vi "mod_Rayleigh Selective Fading (Gans).vi"(0 "profile length (samples)":i32=1000, 1 "number of paths":i32, 5 "sampling frequency (Hz)":dbl=1.0 format="%.2f", 7 "doppler spread (Hz)":dbl=0.01 format="%.2p", 9 "seed in (0xFFFFFFFF)":i32=-1 format="%.0x", 11 "error in (no error)":errorcluster, 12 "fading variance":dbl=1.0 format="%.2f", 13 "reset? (T)":bool=TRUE) -> (4 "Rayleigh fading profile":cdb[][](array[numeric]), 10 "seed out":i32 format="%.0x", 15 "error out":errorcluster)   [LabVIEW 2020, in "niDMT.lvlib"]
doc: "The Rayleigh fading channel is generated based on Clarke and Gans Model using the Doppler filter with U-shaped power spectral density. \n \n\n Inputs:\n 1) Doppler spread (Hz) \n - range : double precision (default:20)\n - an example : a running vehicle with 65mph (104km/h), the carrier frequency of 900MHz\n The speed of the vehicle = 65*1.6*1000/3600 = 28.89m/s\n Doppler frequency = (900MHz)*(28.89m/s)/(300*10^6m/s) = 86.67 Hz\n 2) Fading variance : the variance of the fading channel output\n - range : double precision (default:2)\n 3) Input waveform : Input signal samples\n - some default values were set.\n (dt:0.00025, the number of samples:4000)\n 4) seed in (0xFFFFFFFF)\n 5) Error in\n\n Outputs:\n 1) Rayleigh fading profile : the complex fading channel output\n 2) Error out"
uses:
  <vilib>/addons/Modulation/niDMT.lvlib
  <vilib>/addons/Modulation/niAMT.lvlib
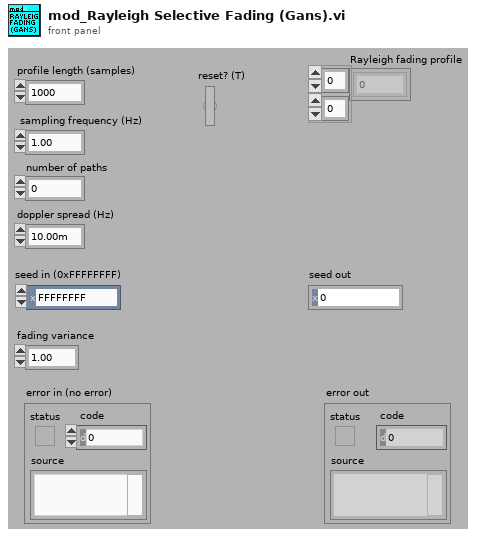
[diagram p1: front panel]
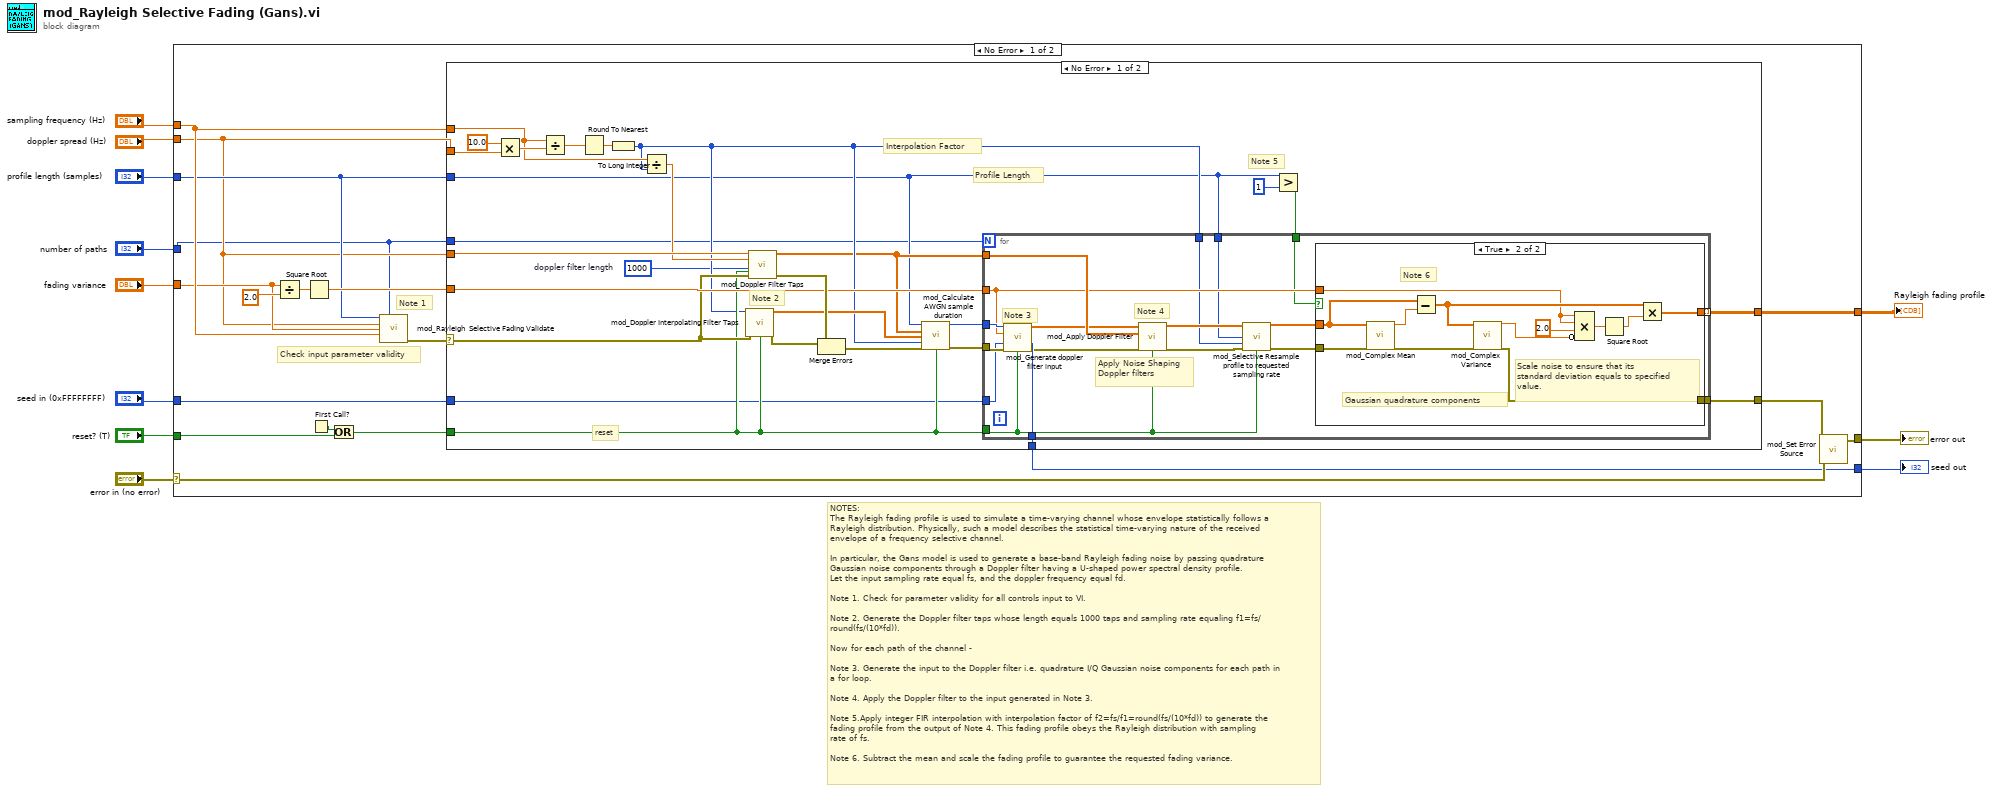
[diagram p0: block diagram]
diagram:
  # "NOTES:\nThe Rayleigh fading profile is used to simulate a time-varying channel whose envelope statistically follows a Rayleigh distribution. Physically, such a model describes the statistical time-varying nature of the received envelope of a frequency selective channel.\n\t\t  \nIn particular, the Gans model is used to generate a base-band Rayleigh fading noise by passing quadrature Gaussian noise components through a Doppler filter having a U-shaped power spectral density profile. \nLet the input sampling rate equal fs, and the doppler frequency equal fd.\n\nNote 1. Check for parameter validity for all controls input to VI.\n\nNote 2. Generate the Doppler filter taps whose length equals 1000 taps and sampling rate equaling f1=fs/round(fs/(10*fd)).\n\nNow for each path of the channel -\n\nNote 3. Generate the input to the Doppler filter i.e. quadrature I/Q Gaussian noise components for each path in a for loop.\n\nNote 4. Apply the Doppler filter to the input generated in Note 3.\n\nNote 5.Apply integer FIR interpolation with interpolation factor of f2=fs/f1=round(fs/(10*fd)) to generate the fading profile from the output of Note 4. This fading profile obeys the Rayleigh distribution with sampling\nrate of fs. \n\nNote 6. Subtract the mean and scale the fading profile to guarantee the requested fading variance."
  n1 = case shown="No Error" "error in (no error)" {
    selector: "error in (no error)" -> [w27 w91]
    tunnel: [w28 w91] -> w11
    tunnel: [w29 _] -> w2
    tunnel: "sampling frequency (Hz)" -> [w19 _]
    tunnel: "doppler spread (Hz)" -> [w14 _]
    tunnel: "fading variance" -> [w18 _]
    tunnel: "profile length (samples)" -> [w17 _]
    tunnel: "seed in (0xFFFFFFFF)" -> [w16 _]
    tunnel: "reset? (T)" -> [w15 _]
    tunnel: [w13 _] -> w3
    tunnel: "number of paths" -> [w12 _]
    frame No Error {
      # "Note 1"
      # "Check input parameter validity"
      n2 = Divide(x=w18, y=2.0) -> (x/y=w22:dbl)
      n3 = Square Root(x=w22) -> (sqrt(x)=w24:dbl)
      n4 = First Call?() -> (First Call?: T/F=w23:bool)
      n5 = Or(x=w23, y=w15) -> (x .or. y?=w20:bool)
      n6 = call <vilib>:"mod_Rayleigh  Selective Fading Validate.vi"("profile length (samples)"=w17, "paths"=w12, "doppler spread (Hz)"=w14, "fading variance"=w18, "sampling frequency"=w19) -> ("error out"=w25:errorcluster)  [unwired: 10 out]
      n7 = case shown="No Error" w25 {
        selector: w25 -> [w39 w90]
        tunnel: [w57 _] -> w29
        tunnel: w14 -> [w55 _]
        tunnel: w17 -> [w31 _]
        tunnel: w24 -> [w42 _]
        tunnel: [w56 w90] -> w26
        tunnel: w20 -> [w36 _]
        tunnel: w16 -> [w33 _]
        tunnel: w19 -> [w48 _]
        tunnel: w14 -> [w50 _]
        tunnel: [w54 _] -> w13
        tunnel: w12 -> [w30 _]
        frame No Error {
          w32 = 1000  # doppler filter length
          # "Interpolation Factor"
          # "Profile Length"
          # "Note 5"
          # "Note 2"
          # "reset"
          n8 = Multiply(x=10.0, y=w50) -> (x*y=w49:dbl)
          n9 = Divide(x=w48, y=w49) -> (x/y=w53:dbl)
          n10 = Round To Nearest(number=w53) -> (nearest integer value=w47:dbl)
          n11 = To Long Integer(number=w47) -> (32bit integer=w35:i32)
          n12 = Divide(x=w48, y=w35) -> (x/y=w52:dbl)
          n13 = call <vilib>:"mod_Doppler Interpolating Filter Taps.vi"("interpolation factor"=w35, "error in (no error)"=w39, "reset? (T)"=w36) -> ("interpolating filter taps"=w37:dbl[], "error out"=w38:errorcluster)  [unwired: 11 out]
          n14 = call <vilib>:"mod_Doppler Filter Taps.vi"("doppler spread (hz)"=w55, "fs"=w52, "doppler filter length"=w32, "error in (no error)"=w39, "reset? (T)"=w36) -> ("doppler filter taps"=w34:dbl[], "error out"=w46:errorcluster)  [unwired: 1 in, 8 out]
          n15 = Merge Errors(w38, w46) -> (w45:errorcluster)
          n16 = call <vilib>:"mod_Calculate AWGN sample duration.vi"("profile length (samples)"=w31, "doppler filter taps"=w34, "interpolating filter taps"=w37, "interpolation factor"=w35, "error in (no error)"=w45, "reset? (T)"=w36) -> ("AWGN samples"=w44:i32, "error out"=w43:errorcluster)  [unwired: 8 out]
          n17 = Greater?(x=w31, y=1) -> (0:w40:bool)
          n18 = for {
            N: w30 -> [_]
            tunnel: [w75] -> w57 mode=indexing
            tunnel: [w74] -> w56
            tunnel: [w73] -> w54
            tunnel: w44 -> [w72]
            tunnel: w43 -> [w71]
            tunnel: w33 -> [w70]
            tunnel: w36 -> [w59]
            tunnel: w35 -> [w63]
            tunnel: w34 -> [w69]
            tunnel: w42 -> [w68]
            tunnel: w40 -> [w67]
            tunnel: w31 -> [w58]
            # "Note 4"
            # "Note 3"
            # "Apply Noise Shaping Doppler filters"
            n19 = call <vilib>:"mod_Generate doppler filter input.vi"("profile length (samples)"=w72, "standard deviation"=w68, "seed in (0xFFFFFFFF)"=w70, "error in (no error)"=w71, "reset? (T)"=w59) -> ("doppler filter input"=w66:cdb[], "seed out"=w73:i32, "error out"=w65:errorcluster)  [unwired: 3 in, 5 out]
            n20 = call <vilib>:"mod_Apply Doppler Filter.vi"("input samples"=w66, "doppler filter taps"=w69, "error in (no error)"=w65, "reset (T)"=w59) -> ("filtered output"=w64:cdb[], "error out"=w62:errorcluster)  [unwired: 2 in, 8 out]
            n21 = call <vilib>:"mod_Selective Resample profile to requested sampling rate.vi"("doppler filter output"=w64, "profile length (samples)"=w58, "interpolation factor"=w63, "error in (no error)"=w62, "reset? (T)"=w59) -> ("fading profile"=w60:cdb[], "error out"=w61:errorcluster)  [unwired: 9 out]
            n22 = case shown="True" w67 {
              tunnel: [w77 w88] -> w75
              tunnel: [w76 w87] -> w74
              tunnel: w61 -> [w76 w86]
              tunnel: w60 -> [w77 w85]
              tunnel: w68 -> [_ w79]
              frame False {
                # "If requested fading profile duration=1 sample, it is meaningless\nto subtract mean and scale for variance."
              }
              frame True {
                # "Note 6"
                # "Scale noise to ensure that its\nstandard deviation equals to specified\nvalue."
                # "Gaussian quadrature components"
                n23 = call <vilib>:"mod_Complex Mean.vi"("Signal In"=w85, "error in (no error)"=w86) -> ("Mean"=w84:cdb, "error out"=w83:errorcluster)  [unwired: 12 out]
                n24 = Subtract(x=w85, y=w84) -> (x-y=w80:cdb[])
                n25 = call <vilib>:"mod_Complex Variance.vi"("Signal In"=w80, "error in (no error)"=w83) -> ("Variance"=w82:dbl, "error out"=w87:errorcluster)  [unwired: 12 out]
                n26 = Compound Arithmetic op=MULTIPLY(w79, w79, 2.0 ("value"), invert w82) -> (w89:dbl)
                n27 = Square Root(x=w89) -> (sqrt(x)=w78:dbl)
                n28 = Multiply(x=w80, y=w78) -> (x*y=w88:cdb[])
              }
            }
          }
        }
        frame Error {
        }
      }
      n29 = call <vilib>:"mod_Set Error Source.vi"("initial error in (no error)"=w27, "final error in (no error)"=w26) -> ("error out"=w28:errorcluster)  [unwired: 1 in, 2 out]
    }
    frame Error {
    }
  }
  "error out" <- w11
  "seed out" <- w3
  "Rayleigh fading profile" <- w2
